vi "Create.vi"(8 "error in (no error)":errorcluster, 10 "Element":refnum<class "Config Element.lvclass">) -> (0 "error out":errorcluster, 3 "Group out":refnum<class "Group.lvclass">)   [LabVIEW 2020, in "VolatusConfig.lvlib" / "Group.lvclass"]
uses:
  Group.lvclass
  C:/dev/lv20CE/relink/lv-volatus/VolatusConfig/VolatusConfigElement/VolatusConfigElement.lvclass
  lv-cdm/CDM-Config/Config Element/Config Element.lvclass
  VolatusConfigElement/VolatusConfigElement.lvclass
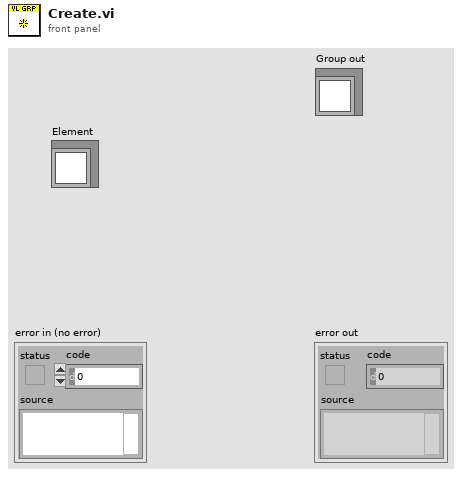
[diagram p1: front panel]
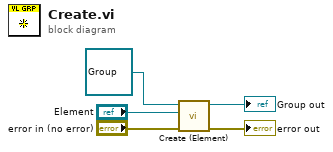
[diagram p0: block diagram]
diagram:
  n1 = call "Create (Element).vi"("error in (no error)"="error in (no error)", "Element"="Element", "VolatusConfigElement in"=refnum<class "Group.lvclass"> refnum ("Group in")) -> ("error out"=→"error out":errorcluster, "VolatusConfigElement out"=→"Group out":refnum<class "Group.lvclass">)  [unwired: 7 in]
